vi "Read Block on Wait.vi"(8 "error in (no error)":errorcluster, 11 "WriteCommand in":refnum<class "WriteCommand.lvclass">) -> (0 "error out":errorcluster, 2 "Block on Wait?":bool, 3 "WriteCommand out":refnum<class "WriteCommand.lvclass">)   [LabVIEW 2023, in "HAF.lvlib" / "WriteCommand.lvclass"]
doc: "Returns whether or not the Command should Block execution whilst it is waiting for other Commands to finish."
uses:
  WriteCommand.lvclass
  WriteCommand.lvclass/WriteCommand.ctl
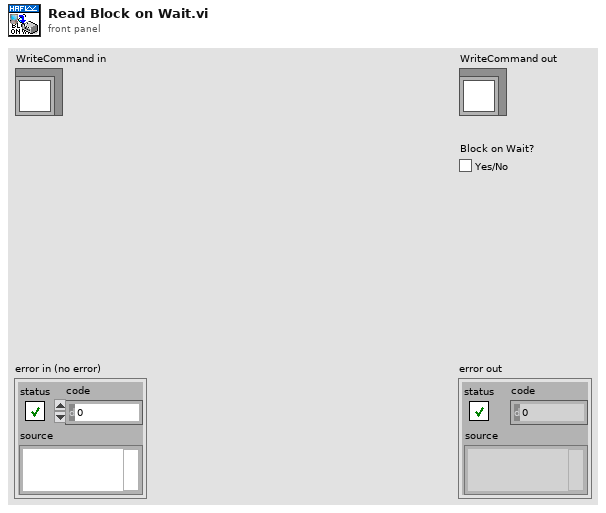
[diagram p1: front panel]
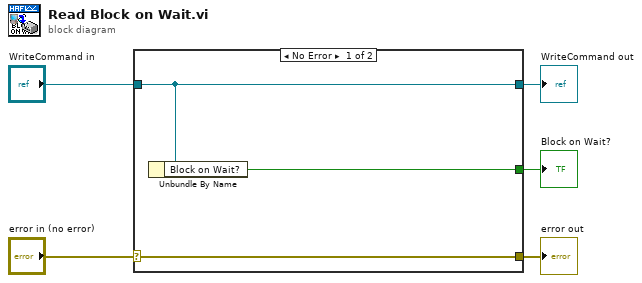
[diagram p0: block diagram]
diagram:
  n1 = case shown="No Error" "error in (no error)" {
    selector: "error in (no error)" -> [w8 w9]
    tunnel: [w8 w9] -> w4
    tunnel: [w7 w10] -> w2
    tunnel: "WriteCommand in" -> [w7 w10]
    tunnel: [w6 _] -> w1
    frame No Error {
      n2 = Unbundle By Name(w7) -> ("Block on Wait?"=w6:bool)
    }
    frame Error {
    }
  }
  "error out" <- w4
  "WriteCommand out" <- w2
  "Block on Wait?" <- w1
